vi "SeCrTs-RPM_Module_A.vi"(7 "Data FIFO Ref":T1, 8 "error in (no error)":errorcluster, 11 "TCP Network Connection in":refnum<k5>) -> (0 "error out":errorcluster, 3 "TCP Network Connection out":refnum<k5>)   [LabVIEW 2022 SP3]
uses:
  RT Support/SeCrTs-RT_Global_R.vi
  RT Controls/SeCrTs-Data FIFO.ctl
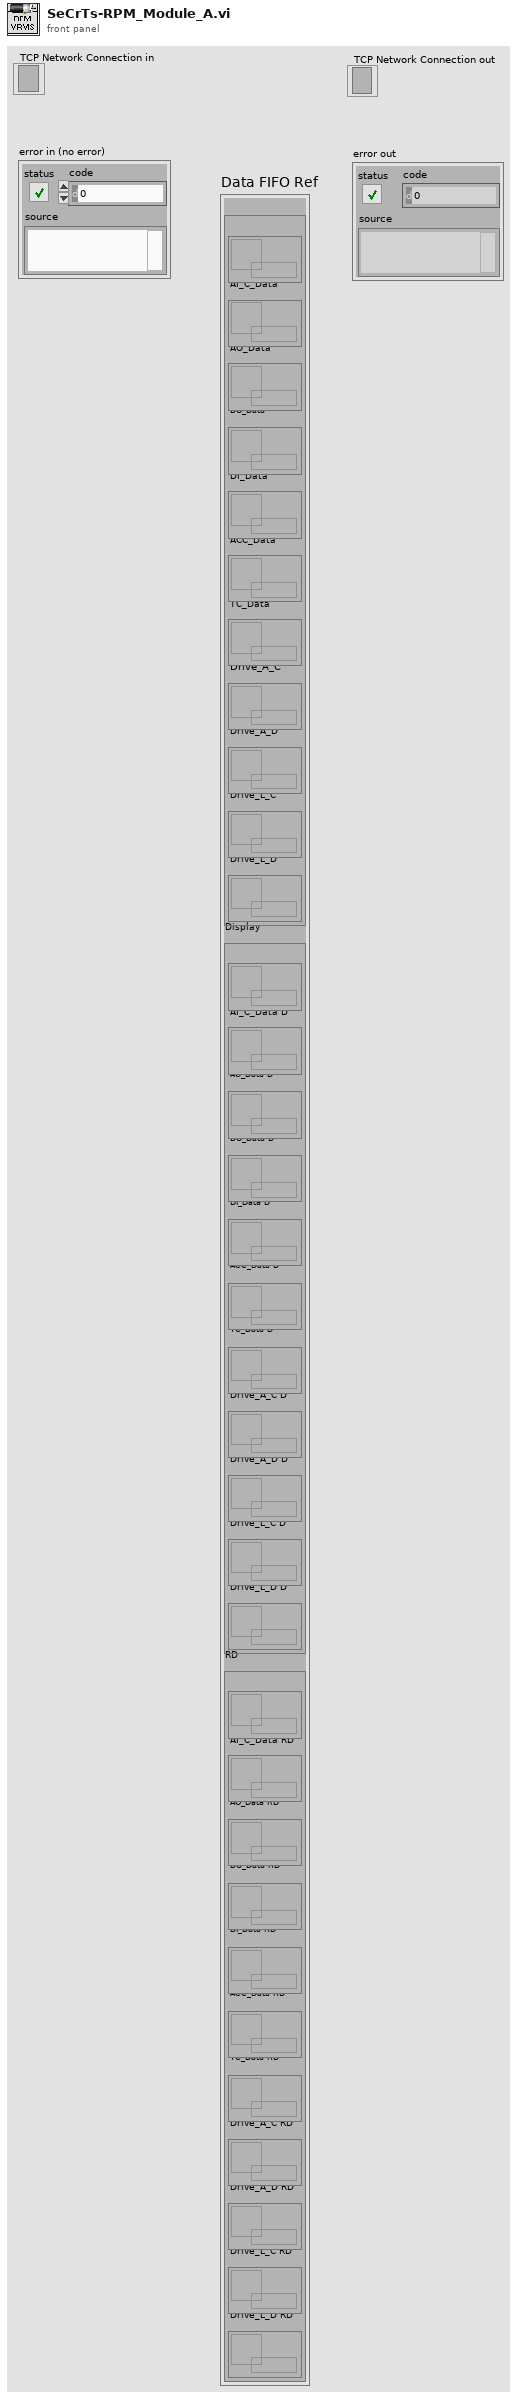
[diagram p1: front panel]
types:
  T1 = typedef "SeCrTs-Data FIFO.ctl" = cluster{"Control":cluster{"AI_V_Data":refnum<queue>, "AI_C_Data":refnum<queue>, "AO_Data":refnum<queue>, "DO_Data":refnum<queue>, "DI_Data":refnum<queue>, "ACC_Data":refnum<queue>, "TC_Data":refnum<queue>, "Drive_A_C":refnum<queue>, "Drive_A_D":refnum<queue>, "Drive_L_C":refnum<queue>, "Drive_L_D":refnum<queue>}, "Display":cluster{"AI_V_Data D":refnum<queue>, "AI_C_Data D":refnum<queue>, "AO_Data D":refnum<queue>, "DO_Data D":refnum<queue>, "DI_Data D":refnum<queue>, "ACC_Data D":refnum<queue>, "TC_Data D":refnum<queue>, "Drive_A_C D":refnum<queue>, "Drive_A_D D":refnum<queue>, "Drive_L_C D":refnum<queue>, "Drive_L_D D":refnum<queue>}, "RD":cluster{"AI_V_Data RD":refnum<queue>, "AI_C_Data RD":refnum<queue>, "AO_Data RD":refnum<queue>, "DO_Data RD":refnum<queue>, "DI_Data RD":refnum<queue>, "ACC_Data RD":refnum<queue>, "TC_Data RD":refnum<queue>, "Drive_A_C RD":refnum<queue>, "Drive_A_D RD":refnum<queue>, "Drive_L_C RD":refnum<queue>, "Drive_L_D RD":refnum<queue>}}
  T2 = enum16{"Standard", "Buffered", "CRLF", "Immediate"}
  T3 = cluster{"En_Drive_A":bool, "En_Drive_L":bool, "Exit_Drive_A":bool, "Exit_Drive_L":bool}
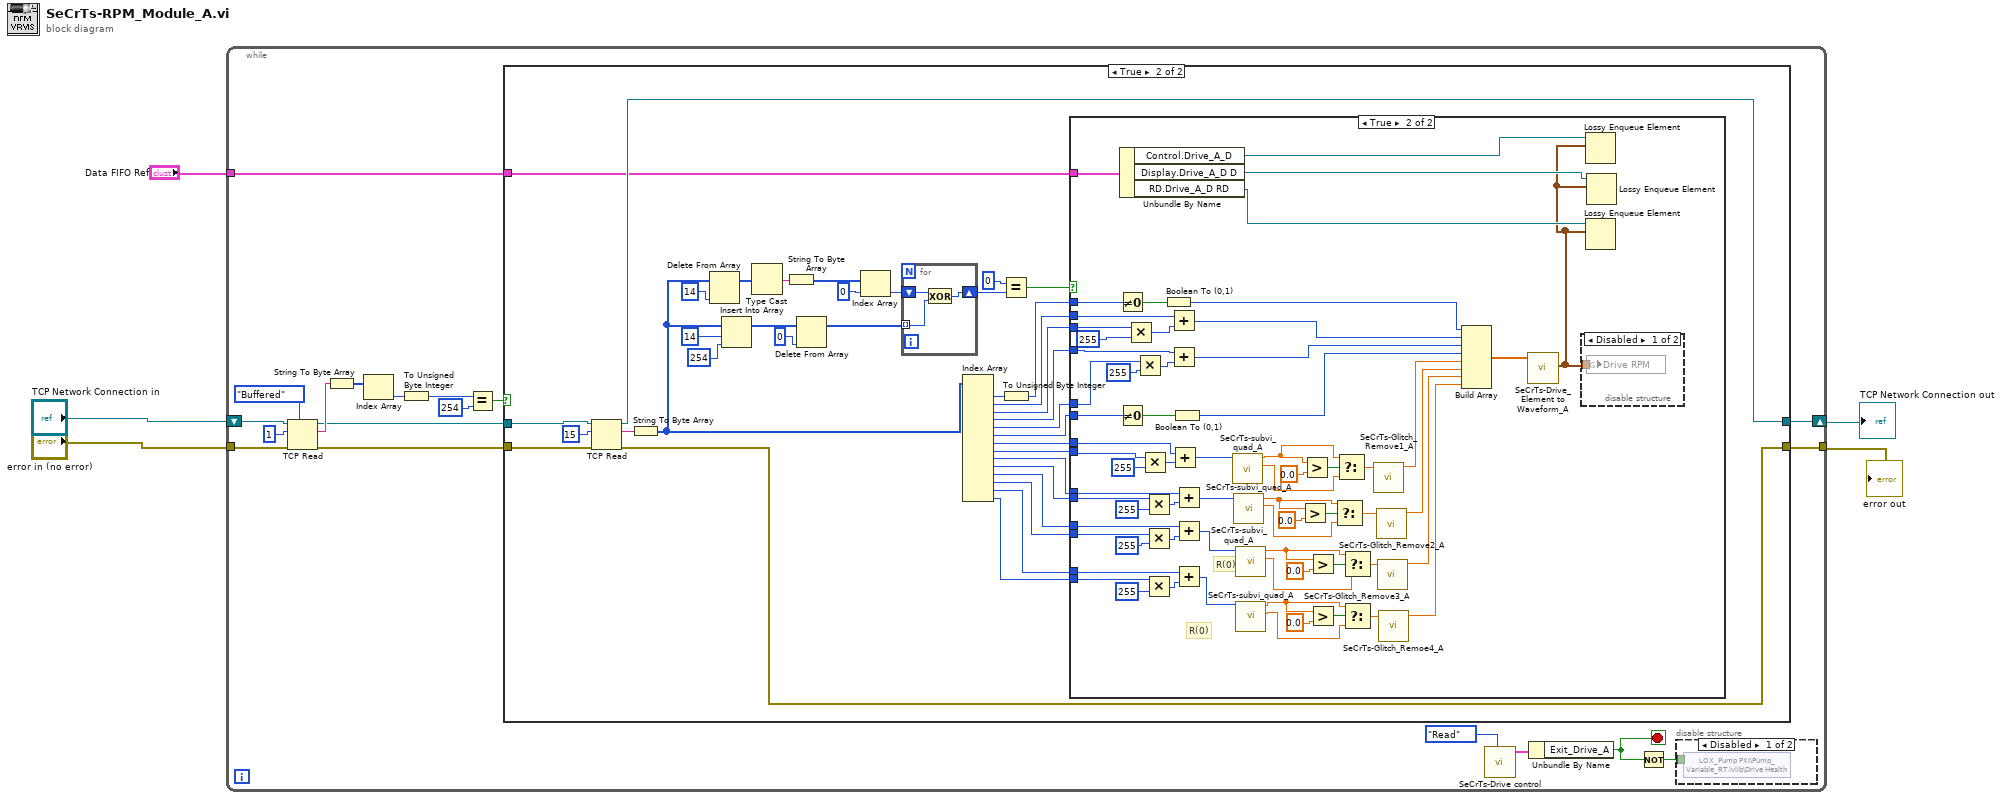
[diagram p0: block diagram]
diagram:
  n1 = while {
    tunnel: "error in (no error)" -> [w23]
    shift-right: [w12] -> w5
    shift-left: "TCP Network Connection in" -> [w24]
    tunnel: [w13] -> w4
    tunnel: "Data FIFO Ref" -> [w6]
    stop <- w7 stop-if-true
    n2 = TCP Read(connection ID=w24, bytes to read=1, error in (no error)=w23, 7:T2."Buffered" ("mode (standard)")) -> (connection ID out=w16:refnum<k5>, data out=w22:string, error out=w15:errorcluster)  [unwired: 1 in]
    n3 = String To Byte Array(string=w22) -> (unsigned byte array=w21:u8[])
    n4 = Index Array(array=w21) -> (element=w20:u8)  [unwired: 1 in]
    n5 = To Unsigned Byte Integer(number=w20) -> (unsigned 8bit integer=w19:u8)
    n6 = Equal?(x=w19, y=u8 254) -> (x = y?=w17:bool)
    n7 = case shown="True" w17 {
      tunnel: w16 -> [w27 w64]
      tunnel: w15 -> [w26 w63]
      tunnel: [w27 w53] -> w12
      tunnel: [w26 w38] -> w13
      tunnel: w6 -> [_ w28]
      frame False {
      }
      frame True {
        n8 = TCP Read(connection ID=w64, bytes to read=15, error in (no error)=w63) -> (connection ID out=w53:refnum<k5>, data out=w61:string, error out=w38:errorcluster)  [unwired: 2 in]
        n9 = String To Byte Array(string=w61) -> (unsigned byte array=w46:u8[])
        n10 = Delete From Array(array=w46, index=14) -> (array with subset deleted=w59:u8[])  [unwired: 1 in, 1 out]
        n11 = Insert Into Array(array=w46, index=14, new element=u8 254 ("new element/subarray")) -> (w52:u8[])
        n12 = Type Cast(x=w59) -> (*(type *) &x=w58:string)  [unwired: 1 in]
        n13 = String To Byte Array(string=w58) -> (unsigned byte array=w57:u8[])
        n14 = Delete From Array(array=w52, index=0) -> (array with subset deleted=w49:u8[])  [unwired: 1 in, 1 out]
        n15 = Index Array(array=w57, index=0) -> (element=w50:u8)
        n16 = for {
          shift-right: [w133] -> w48
          shift-left: w50 -> [w134]
          tunnel: w49 -> [w132] mode=indexing
          n17 = Exclusive Or(1:w132, 2:w134) -> (0:w133:u8)
        }
        n18 = Index Array(array=w46) -> (element #1=w45:u8, element #2=w43:u8, element #3=w42:u8, element #4=w41:u8, element #5=w40:u8, element #6=w39:u8, element #7=w36:u8, element #8=w35:u8, element #9=w34:u8, element #10=w33:u8, element #11=w32:u8, element #12=w31:u8, element #13=w30:u8, element #14=w29:u8)  [unwired: 14 in]
        n19 = Equal?(x=u8 0, y=w48) -> (x = y?=w47:bool)
        n20 = To Unsigned Byte Integer(number=w45) -> (unsigned 8bit integer=w44:u8)
        n21 = case shown="True" w47 {
          tunnel: w44 -> [_ w130]
          tunnel: w43 -> [_ w98]
          tunnel: w42 -> [_ w97]
          tunnel: w41 -> [_ w96]
          tunnel: w40 -> [_ w95]
          tunnel: w39 -> [_ w126]
          tunnel: w36 -> [_ w117]
          tunnel: w35 -> [_ w116]
          tunnel: w34 -> [_ w115]
          tunnel: w33 -> [_ w114]
          tunnel: w32 -> [_ w113]
          tunnel: w31 -> [_ w112]
          tunnel: w30 -> [_ w111]
          tunnel: w29 -> [_ w110]
          tunnel: w28 -> [_ w70]
          frame False {
          }
          frame True {
            # "R(0)"
            # "R(0)"
            n22 = Not Equal To 0?(x=w130) -> (x != 0?=w101:bool)
            n23 = Not Equal To 0?(x=w126) -> (x != 0?=w100:bool)
            n24 = Unbundle By Name(w70) -> ("Control.Drive_A_D"=w69:refnum<queue>, "Display.Drive_A_D D"=w68:refnum<queue>, "RD.Drive_A_D RD"=w67:refnum<queue>)
            n25 = Multiply(x=w97, y=u32 255) -> (x*y=w99:u32)
            n26 = Multiply(x=w95, y=u32 255) -> (x*y=w127:u32)
            n27 = Multiply(x=w116, y=u32 255) -> (x*y=w118:u32)
            n28 = Multiply(x=w114, y=u32 255) -> (x*y=w121:u32)
            n29 = Multiply(x=w112, y=u32 255) -> (x*y=w122:u32)
            n30 = Multiply(x=w110, y=u32 255) -> (x*y=w125:u32)
            n31 = Boolean To (0,1)(Boolean=w101) -> (0, 1=w94:i16)
            n32 = Add(x=w98, y=w99) -> (x+y=w93:u32)
            n33 = Add(x=w96, y=w127) -> (x+y=w92:u32)
            n34 = Add(x=w117, y=w118) -> (x+y=w90:u32)
            n35 = Boolean To (0,1)(Boolean=w100) -> (0, 1=w91:i16)
            n36 = Add(x=w115, y=w121) -> (x+y=w87:u32)
            n37 = Add(x=w113, y=w122) -> (x+y=w84:u32)
            n38 = Add(x=w111, y=w125) -> (x+y=w81:u32)
            n39 = call "SeCrTs-subvi_quad_A.vi"("input variable"=w90) -> ("output variable 2"=w88:dbl, "output variable"=w89:dbl)  [unwired: 8 in]
            n40 = call "SeCrTs-subvi_quad_A.vi"("input variable"=w87) -> ("output variable 2"=w85:dbl, "output variable"=w86:dbl)  [unwired: 8 in]
            n41 = call "SeCrTs-subvi_quad_A.vi"("input variable"=w84) -> ("output variable 2"=w82:dbl, "output variable"=w83:dbl)  [unwired: 8 in]
            n42 = call "SeCrTs-subvi_quad_A.vi"("input variable"=w81) -> ("output variable 2"=w79:dbl, "output variable"=w80:dbl)  [unwired: 8 in]
            n43 = Greater?(x=w86, y=0.0) -> (0:w104:bool)
            n44 = Greater?(x=w89, y=0.0) -> (0:w102:bool)
            n45 = Greater?(x=w83, y=0.0) -> (0:w106:bool)
            n46 = Greater?(x=w80, y=0.0) -> (0:w108:bool)
            n47 = Select(t=w86, s=w104, f=w85) -> (s? t:f=w72:dbl)
            n48 = Select(t=w89, s=w102, f=w88) -> (s? t:f=w78:dbl)
            n49 = Select(t=w83, s=w106, f=w82) -> (s? t:f=w74:dbl)
            n50 = Select(t=w80, s=w108, f=w79) -> (s? t:f=w76:dbl)
            n51 = call "SeCrTs-Glitch_Remove1_A.vi"("Input"=w78) -> ("Output"=w77:dbl)  [unwired: 10 in]
            n52 = call "SeCrTs-Glitch_Remove2_A.vi"("Input"=w72) -> ("Output"=w71:dbl)  [unwired: 10 in]
            n53 = call "SeCrTs-Glitch_Remove3_A.vi"("Input"=w74) -> ("Output"=w73:dbl)  [unwired: 10 in]
            n54 = call "SeCrTs-Glitch_Remoe4_A.vi"("Input"=w76) -> ("Output"=w75:dbl)  [unwired: 10 in]
            n55 = Build Array(w94, w93, w92, w91, w77, w71, w73, w75) -> (w66:dbl[])
            n56 = call "SeCrTs-Drive_Element to Waveform_A.vi"("Array input"=w66) -> ("RPM out"=w65:waveform(dbl)[])  [unwired: 10 in]
            n57 = disable-structure shown="Disabled" {
              disable-tunnel: w65 -> [w131 _]
              frame Disabled {
                n58 = global write "SeCrTs-RT_Global_R.vi" "Drive RPM"(w131) -> ()
              }
              frame Enabled {
              }
            }
            n59 = Lossy Enqueue Element(queue=w69, element=w65) -> ()  [unwired: 1 in, 4 out]
            n60 = Lossy Enqueue Element(queue=w67, element=w65) -> ()  [unwired: 1 in, 4 out]
            n61 = Lossy Enqueue Element(queue=w68, element=w65) -> ()  [unwired: 1 in, 4 out]
          }
        }
      }
    }
    n62 = call "SeCrTs-Drive control.vi"("Action"=enum16{"Init", "Write", "Read"}."Read") -> ("Loop Control Out"=w8:T3)  [unwired: 9 in, 1 out]
    n63 = Unbundle By Name(w8) -> ("Exit_Drive_A"=w7:bool)
    n64 = Not(x=w7) -> (.not. x?=w10:bool)
    n65 = disable-structure shown="Disabled" {
      disable-tunnel: w10 -> [w25 _]
      frame Disabled {
        n66 = shared-variable "LOX_Pump PXI\\Pump_Variable_RT.lvlib\\Drive Health"(w25) -> ()  [unwired: 1 in, 1 out]
      }
      frame Enabled {
      }
    }
  }
  "TCP Network Connection out" <- w5
  "error out" <- w4
